vi "SeqMgr.If Statement, Find Else or End.vi"(9 "Arguements":string[](array[string]), 10 "Next Step":i32, 11 "Sequence":string[][](array[string])) -> (0 "error out":errorcluster, 2 "Next Step":i32, 3 "End":bool)   [LabVIEW 2024, in "EQMF.lvlib" / "SeqMgr.lvlib"]
uses:
  SeqMgr.lvlib
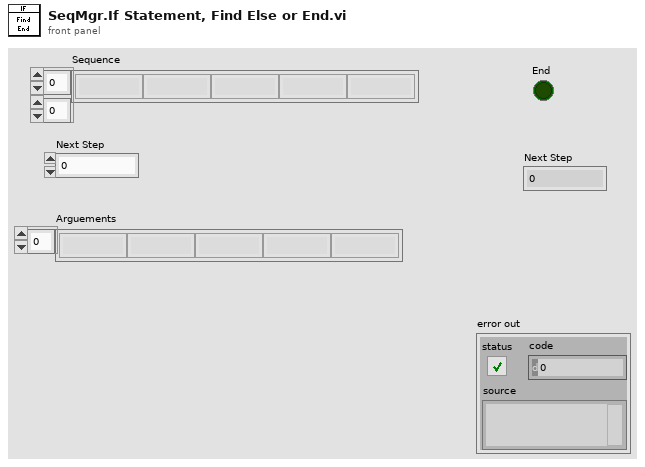
[diagram p1: front panel]
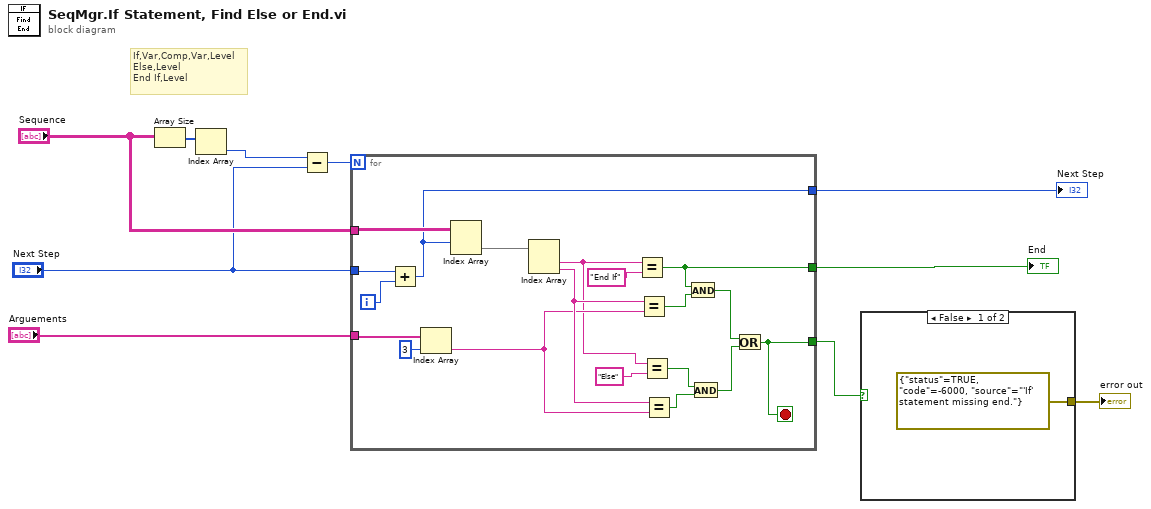
[diagram p0: block diagram]
diagram:
  # "If,Var,Comp,Var,Level\nElse,Level\nEnd If,Level"
  n1 = Array Size(array="Sequence") -> (size(s)=w7:i32[])
  n2 = Index Array(array=w7) -> (element=w2:i32)  [unwired: 1 in]
  n3 = Subtract(x=w2, y="Next Step") -> (x-y=w6:i32)
  n4 = for {
    N: w6 -> [_]
    tunnel: "Next Step" -> [w29]
    tunnel: "Sequence" -> [w27]
    tunnel: "Arguements" -> [w24]
    tunnel: [w16] -> w9
    tunnel: [w13] -> w3
    tunnel: [w11] -> w4
    i -> [w28]
    stop <- w13 stop-if-true
    n5 = Add(x=w29, y=w28) -> (x+y=w16:i32)
    n6 = Index Array(array=w24, index=3) -> (element=w17:string)
    n7 = Index Array(array=w27, index (row)=w16) -> (element=w26:string[])  [unwired: 1 in]
    n8 = Index Array(array=w26) -> (element #1=w12:string, element #2=w18:string)  [unwired: 2 in]
    n9 = Equal?(x=w12, y="End If") -> (x = y?=w11:bool)
    n10 = Equal?(x=w18, y=w17) -> (x = y?=w21:bool)
    n11 = Equal?(x=w12, y="Else") -> (x = y?=w19:bool)
    n12 = Equal?(x=w18, y=w17) -> (x = y?=w20:bool)
    n13 = And(x=w11, y=w21) -> (x .and. y?=w14:bool)
    n14 = And(x=w19, y=w20) -> (x .and. y?=w15:bool)
    n15 = Or(x=w14, y=w15) -> (x .or. y?=w13:bool)
  }
  "End" <- w4
  "Next Step" <- w9
  n16 = case shown="False" w3 {
    tunnel: [errorcluster {"status"=TRUE, "code"=-6000, "source"="'If' statement missing end."} ("error constant") _] -> w5
    frame False {
    }
    frame True {
    }
  }
  "error out" <- w5
